vi "Initialize Transfer Groups.vi"(8 "error in (no error)":errorcluster, 9 "group status pointers":refnum<class "Status Pointer.lvclass">[](array[class]), 10 "Transfer Groups in":refnum<class "Transfer Group.lvclass">[](array[class]), 11 "Plugin in":refnum<class "Plugin.lvclass">) -> (0 "error out":errorcluster, 2 "Transfer Groups out":refnum<class "Transfer Group.lvclass">[](array[class]), 3 "Plugin out":refnum<class "Plugin.lvclass">)   [LabVIEW 2019, in "DSF Core.lvlib" / "Plugin.lvclass"]
uses:
  Plugin.lvclass
  Transfer Group/Transfer Group.lvclass
  Status/Status Pointer.lvclass
  C:/Program Files (x86)/National Instruments/LabVIEW 2019/vi.lib/NI/Memory Manager/Classes/Pointer/Pointer.lvclass
  Plugin.lvclass/Plugin.ctl
  Timing/Timing.lvclass/Timing.ctl
  <vilib>/NI/Memory Manager/Classes/Pointer/Pointer.lvclass/Pointer.ctl
  Transfer Group/Transfer Group.lvclass/Transfer Group.ctl
  Transfer/Transfer.lvclass/Transfer.ctl
  <vilib>/NI/Memory Manager/Classes/Pointer/Is Null.vi
  Status/Create.vi
  Transfer Group/Sort by Priority.vi
  Transfer Group/Separate Rx and Tx.vi
  Transfer Group/Separate Inline and Async.vi
  <vilib>/NI/Memory Manager/Classes/Pointer/Get Address.vi
  <vilib>/NI/Memory Manager/Classes/Pointer/Allocate.vi
  Status/Status Size.vi
  Status/Write Status 1D.vi
  Transfer Group/Get Direction.vi
  Transfer Group/Get Timing.vi
  Transfer Group/Set Active.vi
  <vilib>/NI/Memory Manager/Classes/Pointer/Set Address.vi
  <vilib>/NI/Memory Manager/Classes/Pointer/Set Size.vi
  <vilib>/NI/Memory Manager/Classes/Pointer/Set Internal.vi
  <vilib>/NI/Memory Manager/Classes/Pointer/Check Size.vi
  <vilib>/NI/Memory Manager/Classes/Pointer/Check Null Pointer.vi
  <vilib>/NI/Memory Manager/Classes/Pointer/Errors.vi
  <vilib>/NI/Memory Manager/Classes/Pointer/Out of Bounds.vi
  <vilib>/NI/Memory Manager/Classes/Pointer/Get Size.vi
  <vilib>/NI/Memory Manager/Classes/Pointer/Null Pointer.vi
  <vilib>/NI/Memory Manager/VIs/Write String to Source.vi
  <vilib>/NI/Memory Manager/Classes/Pointer/Write Pointer Size to Error.vi
  <vilib>/NI/Memory Manager/Classes/Pointer/Create Error.vi
  <vilib>/NI/Memory Manager/VIs/Write Numeric to Source.vi
  <vilib>/NI/Memory Manager/VIs/Write Numeric Scalar to Source (Base10 U64).vi
  <vilib>/NI/Memory Manager/VIs/New Error Cluster.vi
  <vilib>/NI/Memory Manager/VIs/New Error Cluster (512B).vi
  <vilib>/NI/Memory Manager/VIs/Set Error Status.vi
  <vilib>/NI/Memory Manager/VIs/Set Error Code.vi
  <vilib>/NI/Memory Manager/VIs/Set Error Source.vi
  <vilib>/NI/Memory Manager/Constants/Constants.vi
  <vilib>/NI/Memory Manager/Constants/Library Name.vi
  <vilib>/NI/Memory Manager/Classes/Pointer/Pointer Error Info.vi
  <vilib>/NI/Memory Manager/Constants/Pointer Class Name.vi
  Timing/Timing.lvclass
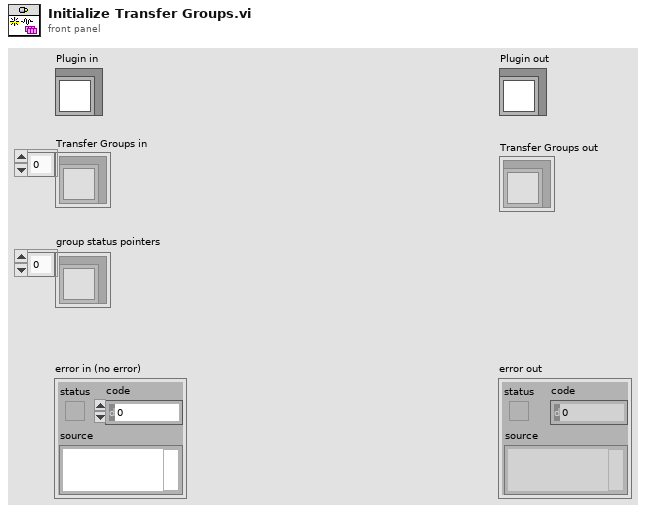
[diagram p1: front panel]
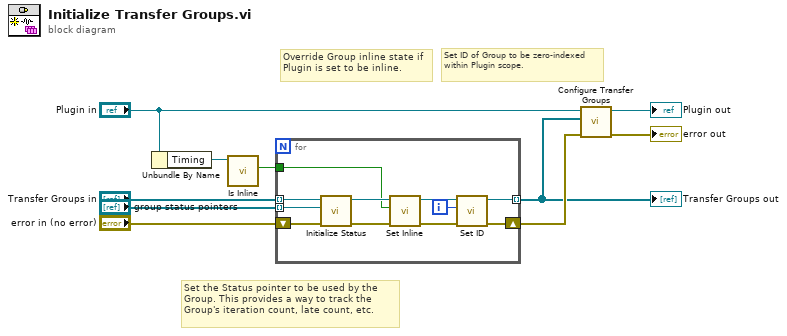
[diagram p0: block diagram]
diagram:
  # "Set the Status pointer to be used by the Group. This provides a way to track the Group's iteration count, late count, etc."
  # "Override Group inline state if Plugin is set to be inline."
  # "Set ID of Group to be zero-indexed within Plugin scope."
  n1 = Unbundle By Name("Plugin in") -> ("Timing"=w6:refnum<class "Timing.lvclass">)
  n2 = call "Is Inline.vi"("Timing in"=w6) -> ("inline?"=w7:bool)  [unwired: 9 in, 1 out]
  n3 = for {
    shift-right: [w17] -> w8
    shift-left: "error in (no error)" -> [w19]
    tunnel: "Transfer Groups in" -> [w18] mode=indexing
    tunnel: w7 -> [w14]
    tunnel: "group status pointers" -> [w15] mode=indexing
    tunnel: [w12] -> w1 mode=indexing
    i -> [w11]
    n4 = call "Initialize Status.vi"("error in (no error)"=w19, "Transfer Group Status"=w15, "Transfer Group in"=w18) -> ("error out"=w17:errorcluster, "Transfer Group out"=w16:refnum<class "Transfer Group.lvclass">)  [unwired: 7 in]
    n5 = call "Set Inline.vi"("inline"=w14, "Transfer Group in"=w16) -> ("Transfer Group out"=w13:refnum<class "Transfer Group.lvclass">)  [unwired: 9 in]
    n6 = call "Set ID.vi"("id"=w11, "Transfer Group in"=w13) -> ("Transfer Group out"=w12:refnum<class "Transfer Group.lvclass">)  [unwired: 9 in]
  }
  "Transfer Groups out" <- w1
  n7 = call "Configure Transfer Groups.vi"("error in (no error)"=w8, "Transfer Groups"=w1, "Plugin in"="Plugin in") -> ("error out"=→"error out":errorcluster, "Plugin out"=→"Plugin out":refnum<class "Plugin.lvclass">)  [unwired: 7 in]
